vi "AR Drone - Simple Control.vi"() -> ()   [LabVIEW 2014]
doc: "Very simple example showing how to use the base VIs to control the AR Drone."
uses:
  <vilib>/LVH/AR Drone Toolkit/AR Drone.lvlib
panel:
  in  "Control Cluster":T1 {"Yaw Speed" scale=-1.0..1.0; "Vertical Speed" scale=-1.0..1.0; "Pitch" scale=-1.0..1.0; "Roll" scale=-1.0..1.0}
  in  "stop":bool
  in  "Emergency Landing":bool
  in  "Take Off/Land":bool
  in  "Hover":bool
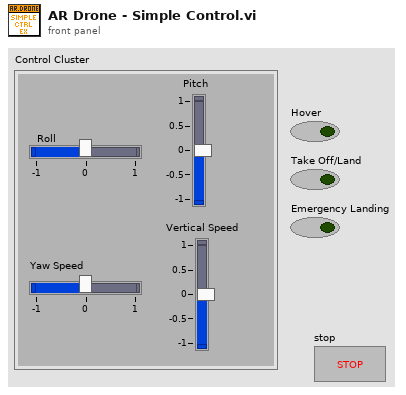
[diagram p1: front panel]
types:
  T1 = cluster{"Roll":sgl, "Pitch":sgl, "Vertical Speed":sgl, "Yaw Speed":sgl}
  T2 = typedef "AR Drone.lvlib/AR Drone Resource.ctl" = cluster{"UDP Control Connection":refnum<k16>, "UDP NavData Connection":refnum<k16>, "UDP Video Connection (Drone 1.0)":refnum<k16>, "TCP Video Connection (Drone 2.0)":refnum<k5>, "TCP Control Port Connection":refnum<k5>, "Drone IP address":string, "Drone Command Port":u16, "Drone NavData Port":u16, "Drone Vid Stream Port":u16, "Drone TCP Control Port":u16, "Home IP address":string, "Home Command Port":u16, "Home NavData Port":u16, "Home Vid Stream Port":u16, "Drone Version":i32}
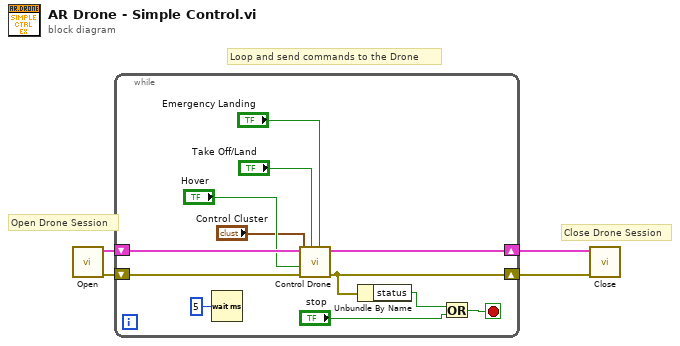
[diagram p0: block diagram]
diagram:
  # "Close Drone Session"
  # "Loop and send commands to the Drone"
  # "Open Drone Session"
  n1 = call <vilib>:"Open.vi"() -> ("error out"=w4:errorcluster, "AR Drone Resource"=w3:T2)  [unwired: 10 in]
  n2 = while {
    shift-right: [w11] -> w2
    shift-left: w3 -> [w15]
    shift-right: [w5] -> w1
    shift-left: w4 -> [w16]
    stop <- w6 stop-if-true
    n3 = Wait (ms)(milliseconds to wait=u32 5) -> ()  [unwired: 1 out]
    n4 = call <vilib>:"Control Drone.vi"("Emergency Landing"="Emergency Landing", "Takeoff/Land"="Take Off/Land", "error in (no error)"=w16, "Hover"="Hover", "Control Cluster"="Control Cluster", "AR Drone Resource"=w15) -> ("error out"=w5:errorcluster, "AR Drone Resource Out"=w11:T2)  [unwired: 4 in]
    n5 = Unbundle By Name(w5) -> ("status"=w8:bool)
    n6 = Or(x=w8, y="stop") -> (x .or. y?=w6:bool)
  }
  n7 = call <vilib>:"Close.vi"("error in (no error)"=w1, "AR Drone Resource"=w2) -> ()  [unwired: 9 in, 1 out]
